vi "ep06_beep_and_pwm_generator.vi"() -> ()   [LabVIEW 2019]
panel:
  in  "%Duty":dbl(knob) scale=0.0..100.0
  in  "stop":bool
  out "Service Status":bool=TRUE
  out "Port Status":bool=TRUE
  out "Information":string="ok: COM3[115200-N-8-1]\r\n"
  in  "Baud Rate":T1(ring)=enum."115200"
  in  "Port Id":T2(ring)=enum."COM3" caption="Port Name"
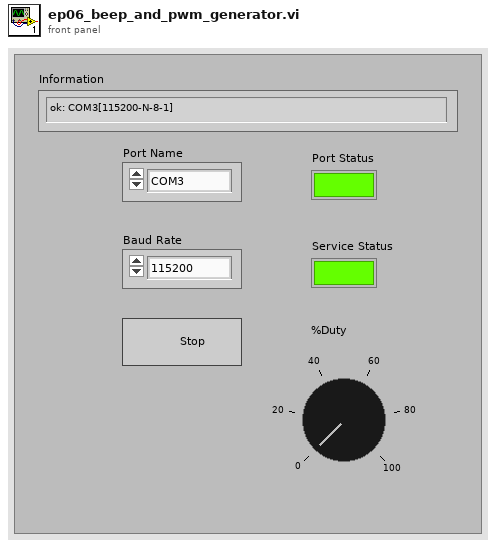
[diagram p1: front panel]
types:
  T1 = enum32{"300", "600", "1200", "2400", "4800", "9600", "14400", "19200", "28800", "38400", "56000", "57600", "115200", "128000", "256000"}
  T2 = enum8{"COM1", "COM2", "COM3", "COM4", "COM5", "COM6", "COM7", "COM8", "COM9", "COM10", "COM11", "COM12", "COM13", "COM14", "COM15", "COM16", "COM17", "COM18", "COM19", "COM20", "COM21", "COM22", "COM23", "COM24", "COM25", "COM26", "COM27", "COM28", "COM29", "COM30", "COM31", "COM32", "COM33", "COM34", "COM35", "COM36", "COM37", "COM38", "COM39", "COM40", "COM41", "COM42", "COM43", "COM44", "COM45", "COM46", "COM47", "COM48"}
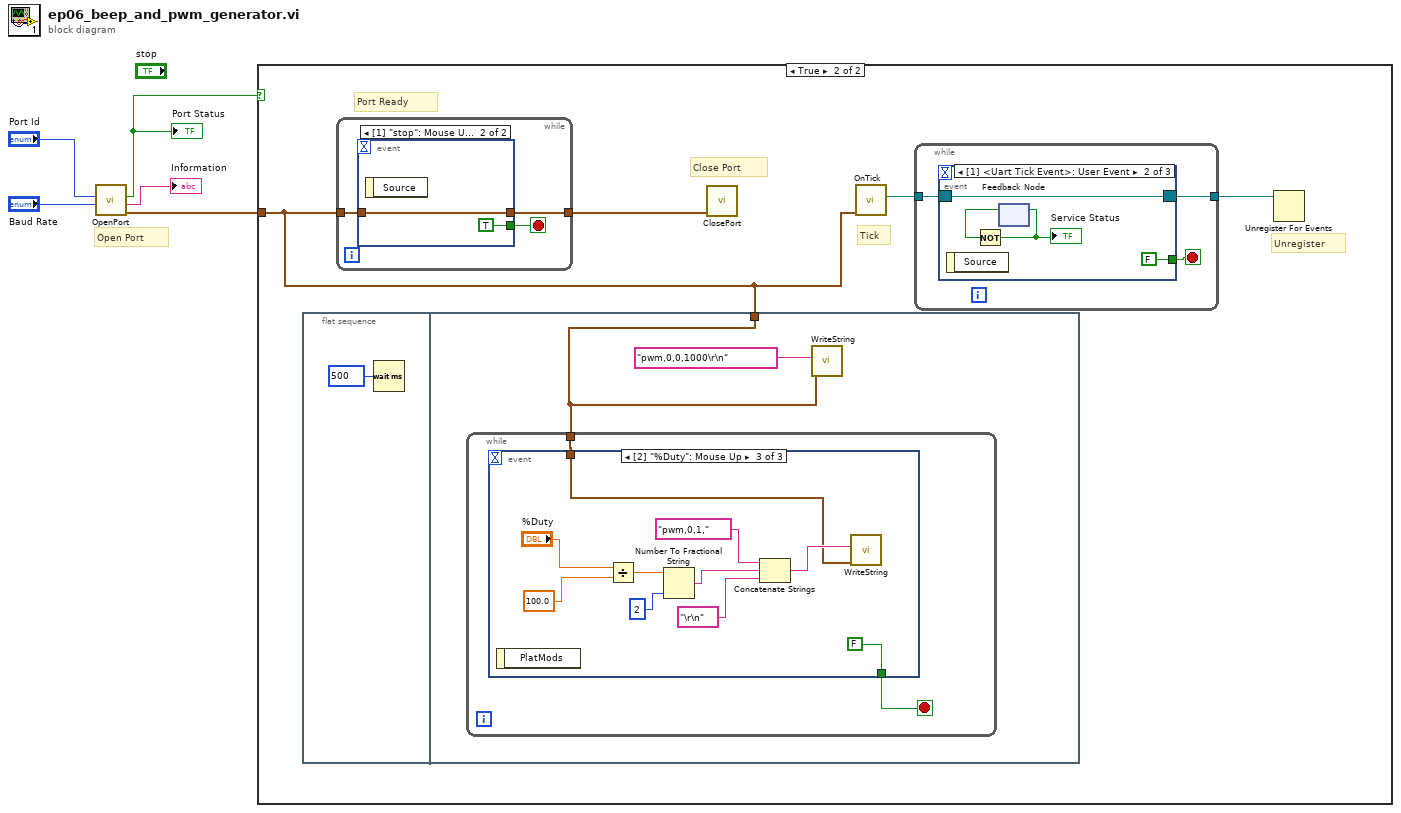
[diagram p0: block diagram]
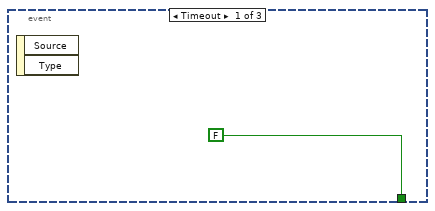
[diagram p3: hidden frame]
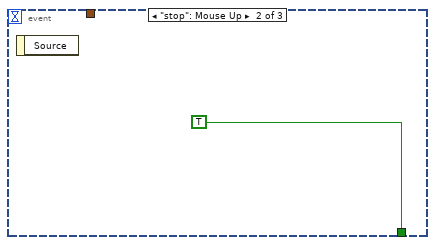
[diagram p4: hidden frame]
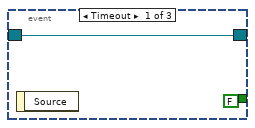
[diagram p5: hidden frame]
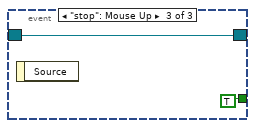
[diagram p6: hidden frame]
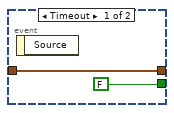
[diagram p7: hidden frame]
diagram:
  # "Open Port"
  n1 = call "OpenPort.vi"("Baud Rate Input"="Baud Rate", "Port Id Input"="Port Id") -> ("Uart Output"=w1:cluster{u64}, "Information"=→"Information":string, "Port Status"=w2:bool)  [unwired: 6 in, 1 out]
  "Port Status" <- w2
  n2 = case shown="True" w2 {
    tunnel: w1 -> [_ w6]
    frame False {
      # "Do nothing"
    }
    frame True {
      # "Unregister"
      # "Close Port"
      # "Tick"
      # "Port Ready"
      n3 = flat-sequence {
        tunnel: w6 -> [w11]
        frame #0 {
          n4 = Wait (ms)(milliseconds to wait=u32 500) -> ()  [unwired: 1 out]
        }
        frame #1 {
          n5 = while {
            tunnel: w11 -> [w13]
            stop <- w14 stop-if-true
            n6 = event shown="[2] \"%Duty\": Mouse Up" {
              selector: _ -> [_ _ _]
              dyn-events: _ -> [_ _ _]
              timeout: _ -> [_ _ _]
              tunnel: [FALSE TRUE FALSE] -> w14
              tunnel: w13 -> [_ _ w19]
              event Timeout {
                n7 = event-data() -> ()  [unwired: 1 in, 2 out]
              }
              event "stop": Mouse Up {
                n8 = event-data() -> ()  [unwired: 1 in, 1 out]
              }
              event "%Duty": Mouse Up {
                n9 = event-data() -> ()  [unwired: 1 in, 1 out]
                n10 = Divide(x="%Duty", y=100.0) -> (x/y=w25:dbl)
                n11 = Number To Fractional String(number=w25, precision (6)=i16 2) -> (F-format string=w26:string)  [unwired: 2 in]
                n12 = Concatenate Strings("pwm,0,1,", w26, "\r\n") -> (w24:string)
                n13 = call "WriteString.vi"("Uart Input"=w19, "String Data"=w24) -> ()  [unwired: 7 in, 3 out]
              }
            }
          }
          n14 = call "WriteString.vi"("Uart Input"=w11, "String Data"="pwm,0,0,1000\r\n") -> ()  [unwired: 7 in, 3 out]
        }
      }
      n15 = while {
        tunnel: w6 -> [w39]
        tunnel: [w38] -> w7
        stop <- w40 stop-if-true
        n16 = event shown="[1] \"stop\": Mouse Up" {
          selector: _ -> [_ _]
          dyn-events: _ -> [_ _]
          timeout: _ -> [_ _]
          tunnel: [FALSE TRUE] -> w40
          tunnel: w39 -> [w41 w43]
          tunnel: [w41 w43] -> w38
          event Timeout {
            n17 = event-data() -> ()  [unwired: 1 in, 1 out]
          }
          event "stop": Mouse Up {
            n18 = event-data() -> ()  [unwired: 1 in, 1 out]
          }
        }
      }
      n19 = call "ClosePort.vi"("Uart Input"=w7) -> ()  [unwired: 9 in, 2 out]
      n20 = call "OnTick.vi"("Uart Input"=w6) -> ("On Tick Event"=w9:refnum<event-registration>)  [unwired: 8 in, 2 out]
      n21 = while {
        tunnel: w9 -> [w28]
        tunnel: [w27] -> w8
        stop <- w29 stop-if-true
        n22 = event shown="[1] <Uart Tick Event>: User Event" {
          selector: w28 -> [w30 w32 w36]
          dyn-events: [w30 w32 w36] -> w27
          timeout: _ -> [_ _ _]
          tunnel: [FALSE FALSE TRUE] -> w29
          event Timeout {
            n23 = event-data() -> ()  [unwired: 1 in, 1 out]
          }
          event User Event {
            n24 = event-data() -> ()  [unwired: 1 in, 1 out]
            n25 = feedback #1() -> (w34:bool)  [unwired: 1 in]
            n26 = Not(x=w34) -> (.not. x?=w33:bool)
            "Service Status" <- w33
            n27 = feedback-in #1(w33) -> ()
          }
          event "stop": Mouse Up {
            n28 = event-data() -> ()  [unwired: 1 in, 1 out]
          }
        }
      }
      n29 = Unregister For Events(event registration refnum=w8) -> ()  [unwired: 1 in, 1 out]
    }
  }
